vi "Write Test Case.lvclass.vi"(8 "error in (no error)":errorcluster, 10 "Test Case.lvclass":refnum<class "Test Case.lvclass">, 11 "Class 1 in":refnum<class "Class 1.lvclass">) -> (0 "error out":errorcluster, 3 "Class 1 out":refnum<class "Class 1.lvclass">)   [LabVIEW 2020, in "Class 1.lvclass"]
uses:
  Class 1.lvclass
  <vilib>/Astemes/LUnit/Test Case.lvclass
  Class 1.lvclass/Class 1.ctl
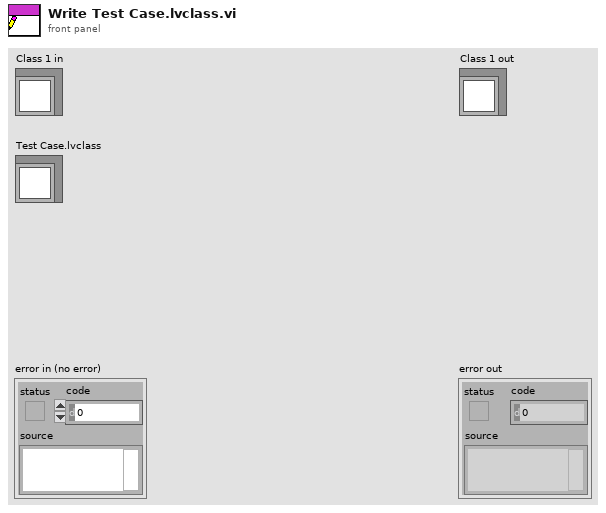
[diagram p1: front panel]
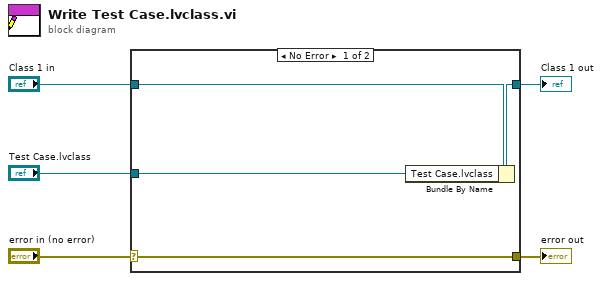
[diagram p0: block diagram]
diagram:
  n1 = case shown="No Error" "error in (no error)" {
    selector: "error in (no error)" -> [w9 w10]
    tunnel: [w9 w10] -> w4
    tunnel: [w7 w11] -> w2
    tunnel: "Class 1 in" -> [w8 w11]
    tunnel: "Test Case.lvclass" -> [w6 _]
    frame No Error {
      n2 = Bundle By Name(cluster=w8, "Test Case.lvclass"=w6) -> (w7:refnum<class "Class 1.lvclass">)
    }
    frame Error {
    }
  }
  "error out" <- w4
  "Class 1 out" <- w2
